vi "Set Default Value.vi"(8 "error in":errorcluster, 10 "Default Value":string, 11 "Object Entry in":refnum<class "Object Entry.lvclass">) -> (0 "error out":errorcluster, 3 "Object Entry out":refnum<class "Object Entry.lvclass">)   [LabVIEW 2020, in "CANopen.lvlib" / "Object Entry.lvclass"]
uses:
  Object Entry.lvclass
  Object Entry.lvclass/Object Entry.ctl
  Sub Object/Sub Object.lvclass
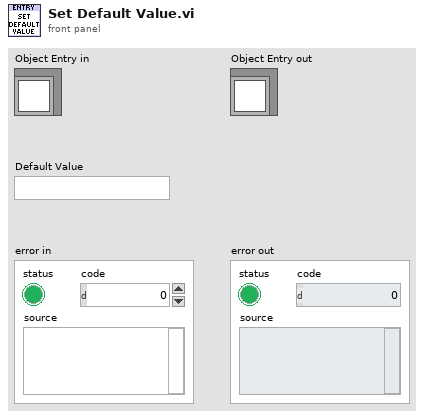
[diagram p1: front panel]
types:
  T1 = typedef "CANopen.lvlib/Object Type.ctl" = u8
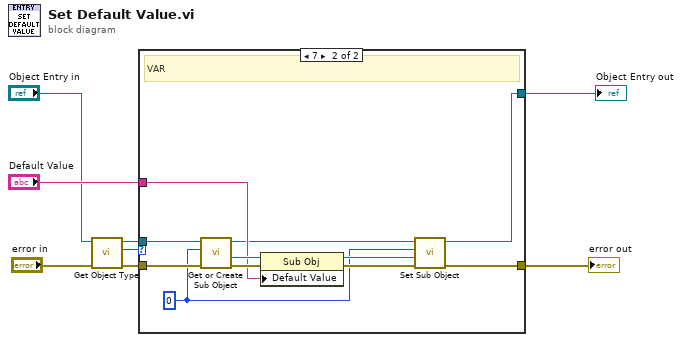
[diagram p0: block diagram]
diagram:
  n1 = call "Get Object Type.vi"("error in"="error in", "Object Entry in"="Object Entry in") -> ("error out"=w2:errorcluster, "Object Type"=w3:T1, "Object Entry out"=w4:refnum<class "Object Entry.lvclass">)  [unwired: 7 in]
  n2 = case shown="7" w3 {
    tunnel: [w9 w13] -> w8
    tunnel: "Default Value" -> [_ w16]
    tunnel: w4 -> [w9 w19]
    tunnel: w2 -> [w10 w21]
    tunnel: [w10 w15] -> w1
    frame Default {
    }
    frame 7 {
      w11 = u8 0 ("Sub Index")
      # "VAR"
      n3 = call "Get or Create Sub Object.vi"("error in"=w21, "Sub Index"=w11, "Obj Entry in"=w19) -> ("error out"=w20:errorcluster, "Sub Object"=w17:refnum<class "Sub Object.lvclass">, "Obj Entry out"=w14:refnum<class "Object Entry.lvclass">)  [unwired: 6 in]
      n4 = property class="Sub Obj"(reference=w17, error in=w20, "Default Value"=w16) -> (reference out=w12:refnum<class "Sub Object.lvclass">, error out=w18:errorcluster)
      n5 = call "Set Sub Object.vi"("error in"=w18, "Sub Object"=w12, "Sub Index"=w11, "Obj Entry in"=w14) -> ("error out"=w15:errorcluster, "Obj Entry out"=w13:refnum<class "Object Entry.lvclass">)  [unwired: 6 in]
    }
  }
  "error out" <- w1
  "Object Entry out" <- w8
